vi "TestGCLabVIEWPython.vi"() -> ()   [LabVIEW 2018]
uses:
  <vilib>/Enthought/Python Integration Toolkit/api/Unpack Double.vi
  <vilib>/Enthought/Python Integration Toolkit/Python Integration Toolkit.lvlib
panel:
  in  "GC folder file name":string
  in  "Result File Name (must include .xlsx)":string
  out "Measured CH4 mol fraction 1":dbl
  out "Measured O2 mol fraction 1":dbl
  out "Measured CO2 mol fraction 1":dbl
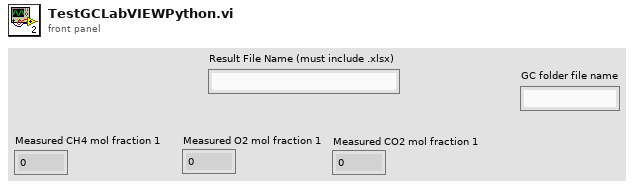
[diagram p1: front panel]
types:
  T1 = typedef "Python Integration Toolkit.lvlib/Session ID.ctl" = u64
  T2 = typedef "Python Integration Toolkit.lvlib/Python Objects.ctl" = variant
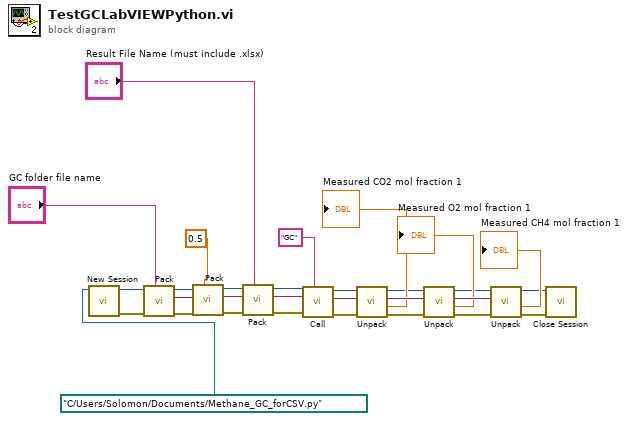
[diagram p0: block diagram]
diagram:
  n1 = call <vilib>:"New Session.vi"("Path to Python Module (.py File)"=path "C:/Users/Solomon/Documents/Methane_GC_forCSV.py") -> ("error out"=w14:errorcluster, "Session ID out"=w12:T1)  [unwired: 9 in]
  n2 = call <vilib>:"Pack.vi"("Argument"="GC folder file name", "error in (no error)"=w14, "Session ID"=w12) -> ("error out"=w17:errorcluster, "Python Object References Out"=w27:T2, "Session ID out"=w16:T1)  [unwired: 6 in]
  n3 = call <vilib>:"Pack.vi"("Argument"=0.5, "error in (no error)"=w17, "Python Object References In"=w27, "Session ID"=w16) -> ("error out"=w8:errorcluster, "Python Object References Out"=w9:T2, "Session ID out"=w10:T1)  [unwired: 5 in]
  n4 = call <vilib>:"Pack.vi"("Argument"="Result File Name (must include .xlsx)", "error in (no error)"=w8, "Python Object References In"=w9, "Session ID"=w10) -> ("error out"=w7:errorcluster, "Python Object References Out"=w6:T2, "Session ID out"=w5:T1)  [unwired: 5 in]
  n5 = call <vilib>:"Call.vi"("Function or Method Name"="GC" ("Function Name"), "error in (no error)"=w7, "Python Object References In"=w6, "Session ID"=w5) -> ("error out"=w21:errorcluster, "Python Object References Out"=w28:T2, "Session ID out"=w18:T1)  [unwired: 5 in]
  n6 = call-poly <vilib>:"Unpack.vi"("error in (no error)"=w21, "Python Object References In"=w28, "Session ID"=w18) -> ("error out"=w22:errorcluster, "Value"=→"Measured CO2 mol fraction 1":dbl, "Python Object References Out"=w29:T2, "Session ID out"=w19:T1)  [unwired: 5 in]
  n7 = call-poly <vilib>:"Unpack.vi"("error in (no error)"=w22, "Python Object References In"=w29, "Session ID"=w19) -> ("error out"=w23:errorcluster, "Value"=→"Measured O2 mol fraction 1":dbl, "Python Object References Out"=w30:T2, "Session ID out"=w20:T1)  [unwired: 5 in]
  n8 = call-poly <vilib>:"Unpack.vi"("error in (no error)"=w23, "Python Object References In"=w30, "Session ID"=w20) -> ("error out"=w15:errorcluster, "Value"=→"Measured CH4 mol fraction 1":dbl, "Session ID out"=w13:T1)  [unwired: 5 in, 1 out]
  n9 = call <vilib>:"Close Session.vi"("error in (no error)"=w15, "Session ID"=w13) -> ()  [unwired: 9 in, 1 out]
